vi "setTargetState.vi"(8 "error in (no error)":errorcluster, 10 "Target State":string, 11 "state in":refnum<class "state.lvclass">) -> (0 "error out":errorcluster, 3 "state out":refnum<class "state.lvclass">)   [LabVIEW 2020, in "eos.lvlib" / "state.lvclass"]
uses:
  state.lvclass
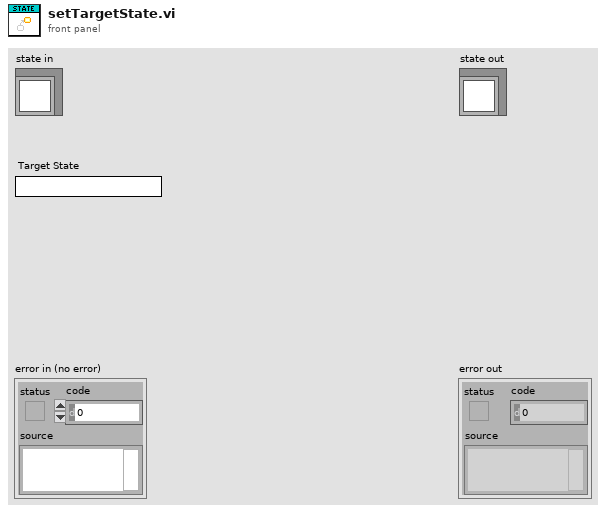
[diagram p1: front panel]
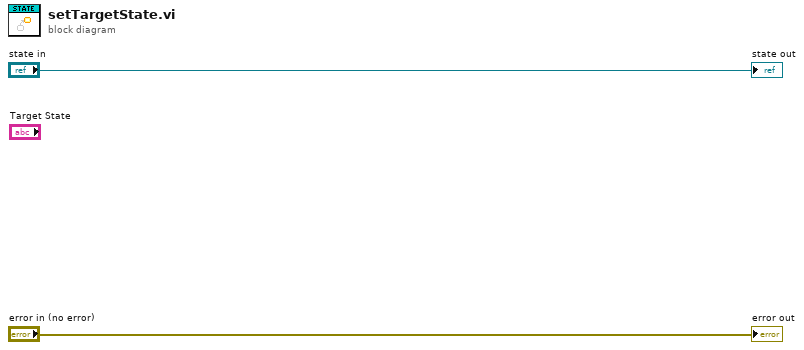
[diagram p0: block diagram]
diagram:
  "error out" <- "error in (no error)"
  "state out" <- "state in"
